vi "Read Channel Settings.vi"(8 "error in (no error)":errorcluster, 11 "FunctionGenerator in":refnum<class "FunctionGenerator.lvclass">) -> (0 "error out":errorcluster, 2 "Settings":T1 {"Fall Time" format="%#_g s"; "Rise Time" format="%#_g s"; "Pulse Width" format="%#_g s"; "Symmetry" format="%#_g %"; "Phase" format="%#_g °"; "Offset" format="%#_g V"; "Amplitude" format="%#_g V"; "Frequency" format="%#_g Hz"}, 3 "FunctionGenerator out":refnum<class "FunctionGenerator.lvclass">)   [LabVIEW 2019, in "FunctionGenerator.lvlib" / "FunctionGenerator.lvclass"]
uses:
  Library/FunctionGenerator.lvclass
  Custom Controls/WaveformSettings.ctl
  Custom Controls/WaveformMode.ctl
  Library/FunctionGenerator.lvclass/FunctionGenerator.ctl
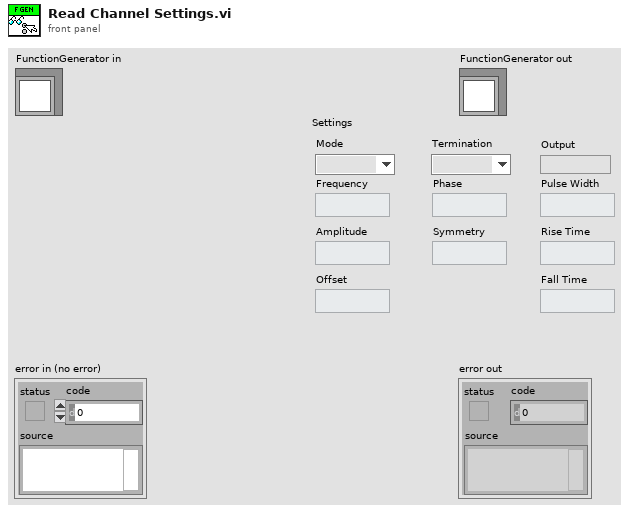
[diagram p1: front panel]
types:
  T1 = typedef "FunctionGenerator.lvlib/FunctionGenerator.lvclass/WaveformSettings.ctl" = cluster{"Frequency":dbl, "Amplitude":dbl, "Offset":dbl, "Phase":dbl, "Symmetry":dbl, "Pulse Width":dbl, "Rise Time":dbl, "Fall Time":dbl, "Mode":T2, "Termination":enum16{"50_Ohm", "High_Z"}, "Output":bool}
  T2 = typedef "FunctionGenerator.lvlib/FunctionGenerator.lvclass/WaveformMode.ctl" = enum16{"Sine", "Square", "Ramp", "Pulse", "Arbitrary", "Triangle", "Noise", "DC"}
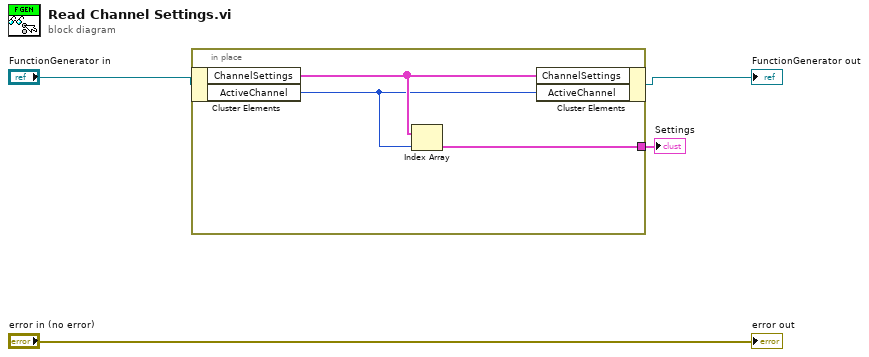
[diagram p0: block diagram]
diagram:
  n1 = in-place {
    in-place-border: [w5] -> w2
    n2 = in-place-cluster #1("FunctionGenerator in") -> ("ChannelSettings"=w7:T1[], "ActiveChannel"=w6:i32)
    n3 = Index Array(array=w7, index=w6) -> (element=w5:T1)
    n4 = in-place-cluster #1("ChannelSettings"=w7, "ActiveChannel"=w6) -> (→"FunctionGenerator out":refnum<class "FunctionGenerator.lvclass">)
  }
  "Settings" <- w2
  "error out" <- "error in (no error)"
